vi "tutorial_02.vi"(1 "Deg C":dbl) -> (0 "Deg F":dbl)   [LabVIEW 2021]
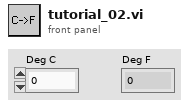
[diagram p1: front panel]
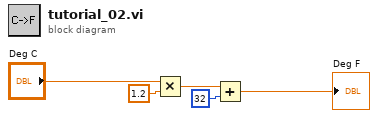
[diagram p0: block diagram]
diagram:
  n1 = Multiply(x="Deg C", y=1.2) -> (x*y=w2:dbl)
  n2 = Add(x=w2, y=32) -> (x+y=→"Deg F":dbl)
